vi "AnnularArraySIR.vi"(0 "Trans Geometry":T5={"ROC (cm)"=1.2, "a (cm)"=0.3, "focus location"=1.2} {"focus location" format="%.2f"; "a (cm)" format="%.2f"; "ROC (cm)" format="%.2f"}, 1 "Pressure Calc":u16(ring)=1 items=["Pos Peak", "Neg peak", "Pk-Pk", "Steady State", "CW Drive", "Pii"], 3 "center of calc":dbl, 4 "Save Options":T3={"Save h Files?"=FALSE, "Save image data?"=FALSE, "Path"=path "F:/Test"}, 5 "Center Hole":dbl format="%.2f", 6 "Recip Processing":u16[][](array[ring])=[[1, 1, 1, 1, 1], [1, 1, 1, 1, 1], [1, 1, 1, 1, 1], [1, 1, 1, 1, 1], [1, 1, 1, 1, 1]] items=["0", "1", "2"], 7 "Wave Source":T1={"Load Wave File"=FALSE, "file path"=path "F:/PVDFXducer/FiveRing/5Ring5/83micH/R1quartz.txt", "Up sample fac"=1}, 8 "Variables":T6={"Number of rings"=5, "sound spd (cm/s)"=150000, "z span (cm)"=0.1, "z steps"=11, "y span (cm)"=0.05, "y steps"=30, "time step (s)"=1e-10, "z"=0.0, "y"=0.0, "ref delay"=0.0, "freq (MHz)"=4.5, "cycles"=5.0} {"freq (MHz)" format="%.2f"; "z span (cm)" format="%.2f"; "y" format="%.2f"; "ref delay" format="%.2f"; "y span (cm)" format="%.4f"; "z" format="%.2f"; "time step (s)" format="%.2e"}, 10 "Calc":u16(ring) items=["One way", "RT Single Rings", "R/T Full Aperture", "Time Domain PSF"], 11 "DR Inputs":T2 {"Tansducer" items=["F2 40 MHz", "F3 20 MHz"]}, 12 "Active Annuli":bool[](array[boolean]), 13 "kerf space (cm)":dbl=0.01 format="%.5f") -> (14 "Output Data":T4 {"pressures" format="%.2f"; "y-axis" format="%.2f"; "z-axis" format="%.2f"}, 19 "time data out":dbl[][](array[numeric]))   [LabVIEW 2022 SP3]
uses:
  <vilib>/Math Plots/3D Math Plots/3D Surface/3D Surface XCtrl/3D Surface.xctl
  <vilib>/Analysis/2dsp.llb/Decimate (single shot, DBL).vi
  <vilib>/Math Plots/3D Math Plots/3D Surface/3D Surface Datatype/Public/Plot Helper (Vector).vi
  <vilib>/Utility/file.llb/Write Delimited Spreadsheet (DBL).vi
  <vilib>/Utility/file.llb/Write To Spreadsheet File (DBL).vi
  <vilib>/Analysis/NI_AALBase.lvlib
  <vilib>/Analysis/NI_AALPro.lvlib
  <vilib>/Math Plots/3D Math Plots/3D Surface/3D Surface Datatype/3D Surface Datatype.lvclass
panel:
  out "3D Surface":refnum<class "3D Plot Datatype.lvclass">[](xcontrol)
  out "data out":sgl[][][](array[numeric])
  out "Waveform Graph":dbl[](graph)
  out "max value":dbl
  in  "norm ?":bool
  in  "Gain":dbl[](array[numeric]) format="%.2f"
  in  "Kerf?":bool=TRUE
  out "3 dB beamwidth axial":dbl format="%.4f"
  in  "SAVE DATA?":bool
  out "oneil axial P":cluster{dbl[], "Y[i]=X[i]/Max|X|":dbl[]}(graph)
  in  "full h(r,t)?":bool
  in  "Number of rings":i32=-1
  in  "Make Report":bool
  out "axial peak (cm)":dbl format="%.2f"
  out "3 dB beamwidth (cm)":dbl format="%.4f"
  out "lateral pressure":cluster{"output":dbl[], "output":dbl[]}(graph)
  out "Rings":picture
  out "axial pressure":cluster{dbl[], "output":dbl[]}(graph)
  # "Quantel Probe\n0 1.895 1.995 2.75 2.85 3.42  3.52  3.99 4.09  4.5 \ngeometricFocusMm=23.2"
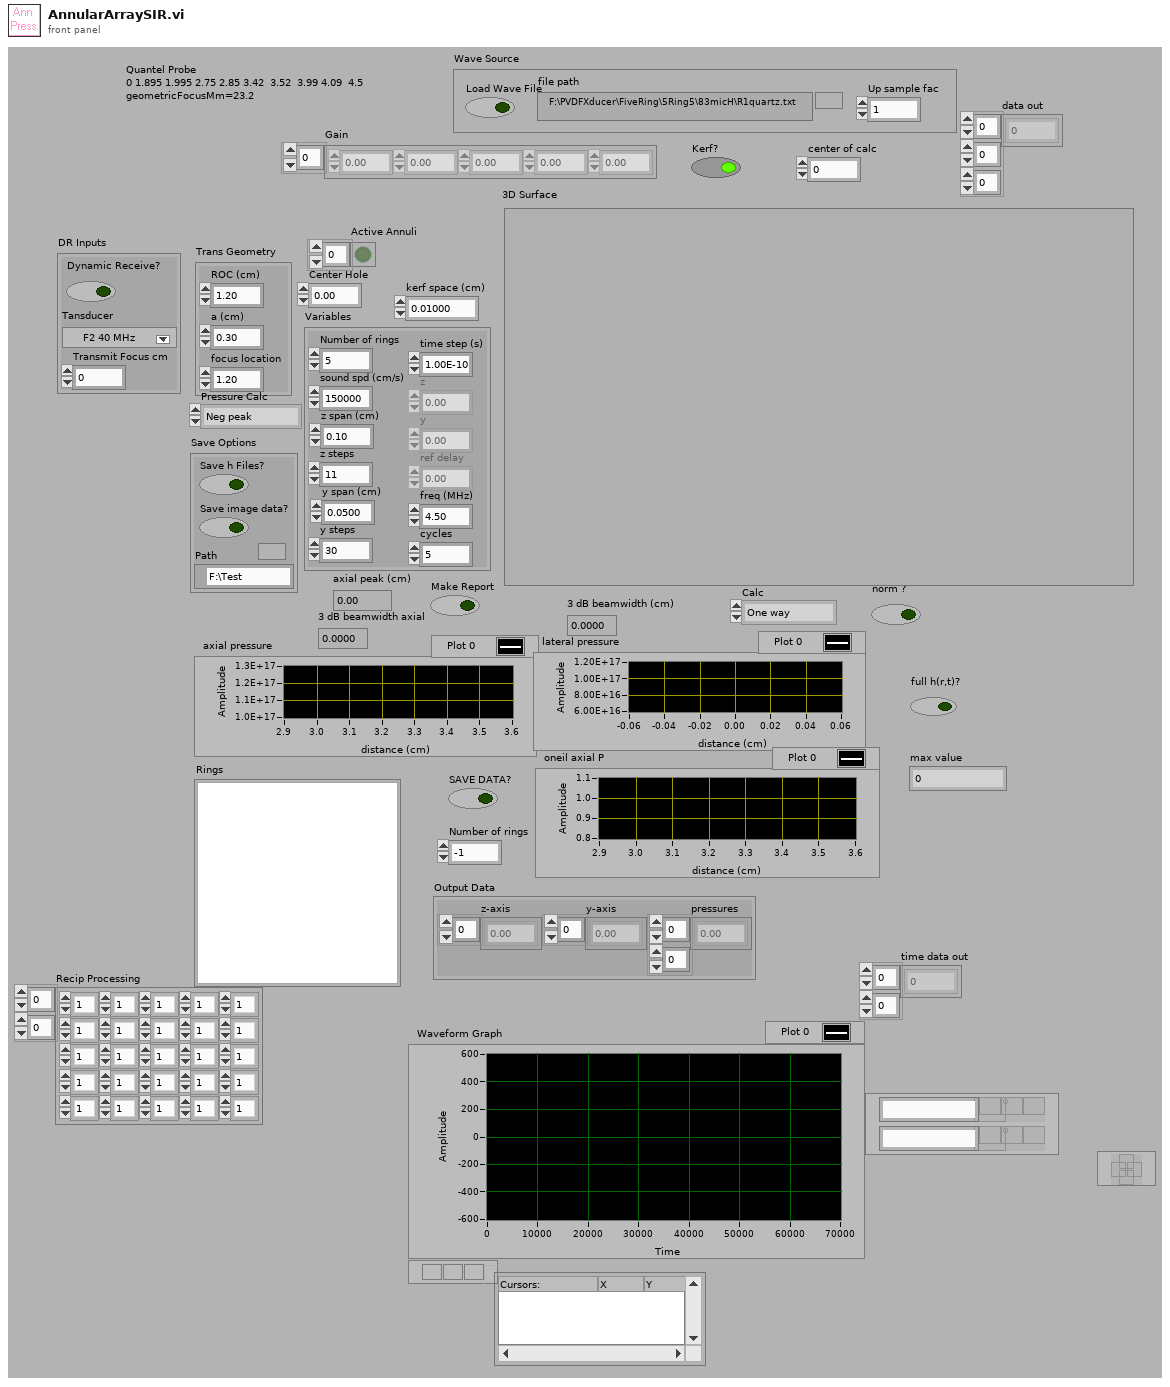
[diagram p1: front panel]
types:
  T1 = cluster{"Load Wave File":bool, "file path":path, "Up sample fac":i32}
  T2 = cluster{"Dynamic Receive?":bool, "Tansducer":u16, "Transmit Focus cm":dbl}
  T3 = cluster{"Save h Files?":bool, "Save image data?":bool, "Path":path}
  T4 = cluster{"z-axis":dbl[], "y-axis":dbl[], "pressures":dbl[][]}
  T5 = cluster{"ROC (cm)":dbl, "a (cm)":dbl, "focus location":dbl}
  T6 = cluster{"Number of rings":i32, "sound spd (cm/s)":i32, "z span (cm)":dbl, "z steps":i32, "y span (cm)":dbl, "y steps":i32, "time step (s)":sgl, "z":dbl, "y":dbl, "ref delay":dbl, "freq (MHz)":dbl, "cycles":sgl}
  T7 = cluster{"Annular rings":cluster{"Radius":dbl, "a":dbl}[], "Waveform":dbl[], "focus delay abs (s)":dbl}[]
  T8 = cluster{"Number of rings":i32, "sound spd (cm/s)":i32, "z span (cm)":dbl, "z steps":i32, "y spacing (cm)":dbl, "y steps":i32, "time step (s)":sgl, "z":dbl, "y":dbl, "ref delay":dbl, "freq (MHz)":dbl, "cycles":sgl}
  T9 = cluster{dbl[], "output":dbl[], "Yij=Xij/Max|X|":dbl[][]}
  T10 = cluster{"axial pressure (z)":cluster{dbl[], "output":dbl[]}, "3 dB beamwidth (cm)":dbl, "lateral pressure (y)":cluster{"output":dbl[], "output":dbl[]}, "3 dB beamwidth (cm)":dbl}
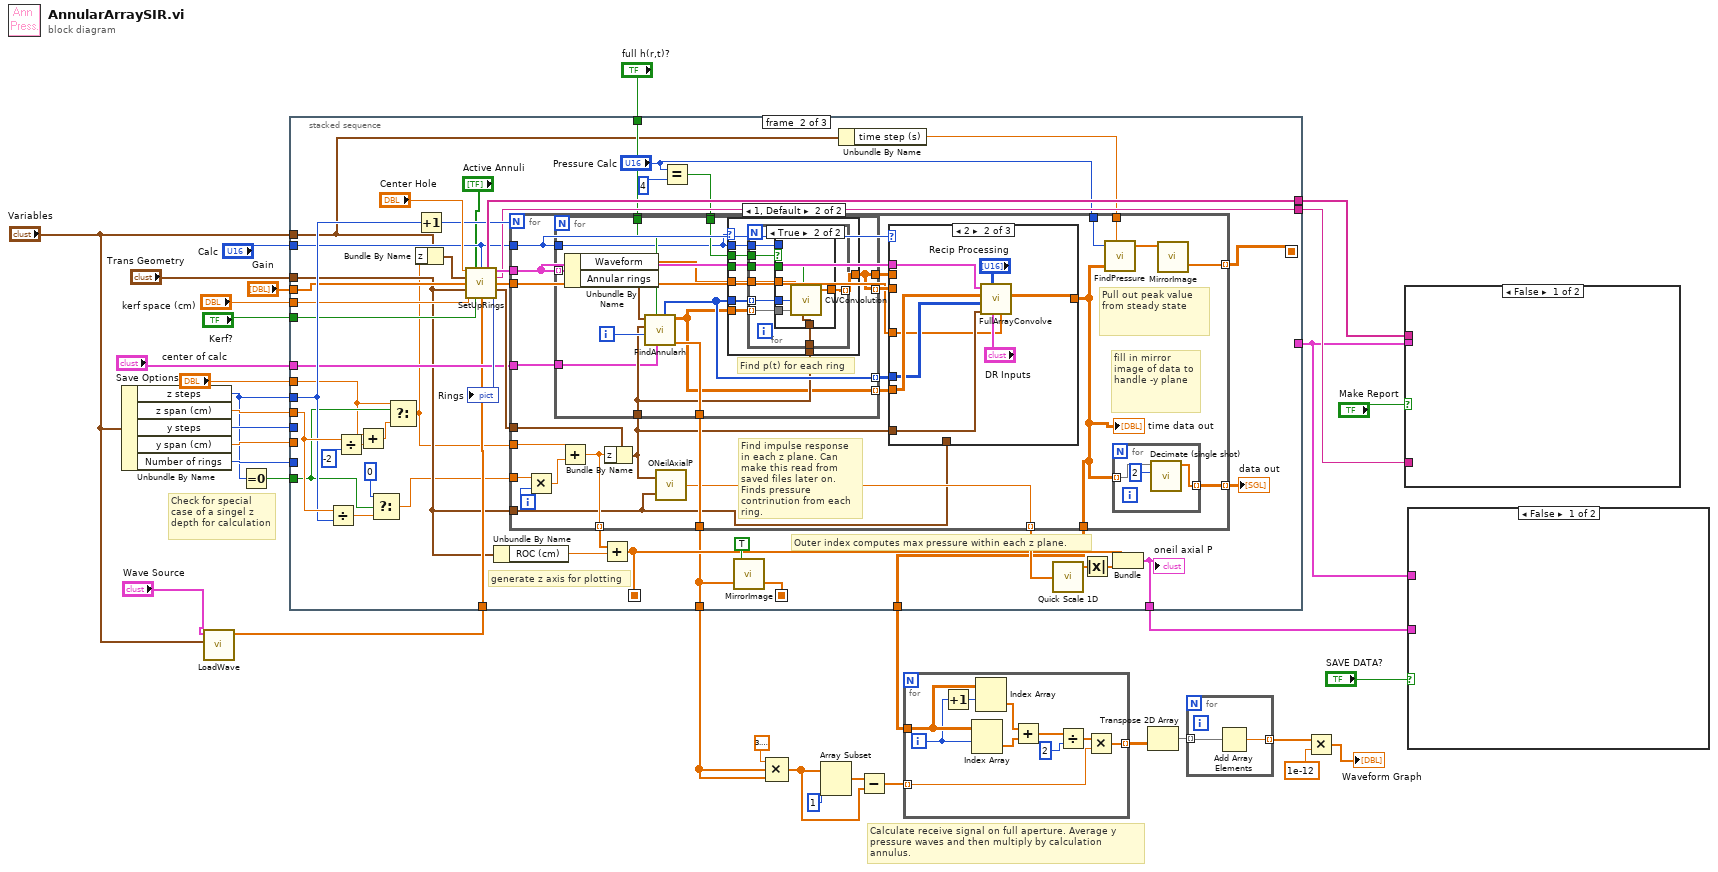
[diagram p0: block diagram]
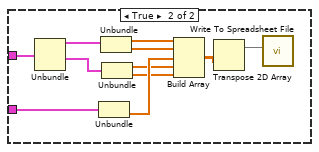
[diagram p2: hidden frame]
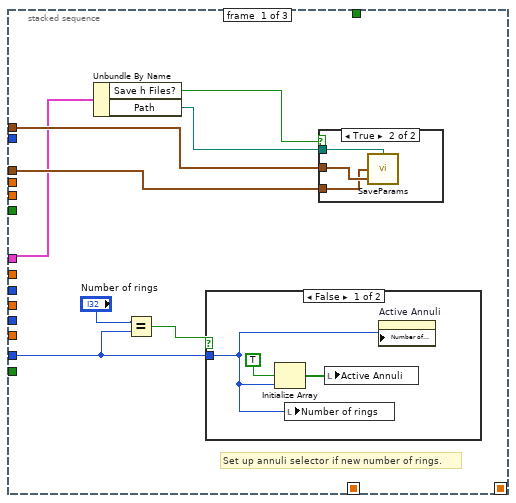
[diagram p3: hidden frame]
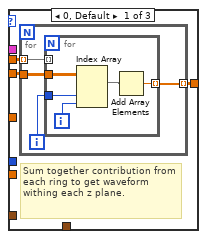
[diagram p6: hidden frame]
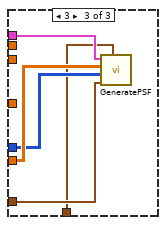
[diagram p7: hidden frame]
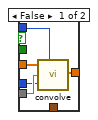
[diagram p9: hidden frame]
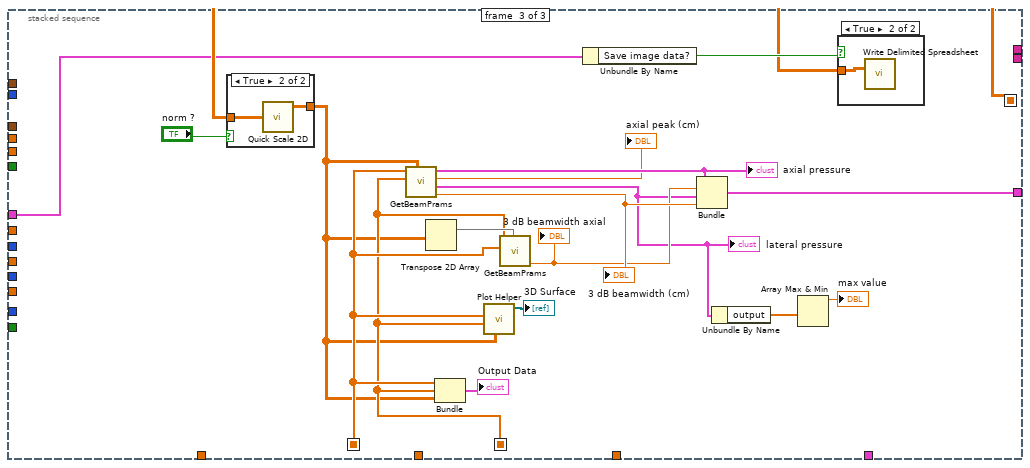
[diagram p10: hidden frame]
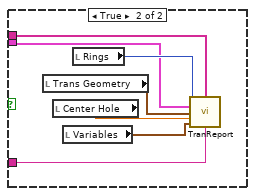
[diagram p13: hidden frame]
diagram:
  # "Calculate receive signal on full aperture. Average y pressure waves and then multiply by calculation annulus."
  # "Check for special case of a singel z depth for calculation"
  n1 = Unbundle By Name("Variables") -> ("z steps"=w17:i32, "z span (cm)"=w35:dbl, "y steps"=w30:i32, "y span (cm)"=w29:dbl, "Number of rings"=w32:i32)
  n2 = call "LoadWave.vi"("Variables"="Variables", "Wave Source"="Wave Source") -> ("Waveform Graph"=w1:dbl[])  [unwired: 1 in, 8 out]
  n3 = Equal To 0?(x=w17) -> (x = 0?=w16:bool)
  n4 = stacked-sequence {
    seq-local: [_ w77 _] -> [_ _ w200]
    seq-local: [_ w84 _] -> [_ _ w192]
    seq-local: [_ w74 _] -> [_ _ w193]
    tunnel: w35 -> [_ w92 _]
    tunnel: "Save Options" -> [w36 w87 w195]
    tunnel: "Trans Geometry" -> [w42 w67 _]
    tunnel: "Variables" -> [w43 w57 _]
    tunnel: w17 -> [_ w88 _]
    tunnel: w32 -> [w38 _ _]
    tunnel: w30 -> [_ _ _]
    tunnel: w29 -> [_ _ _]
    tunnel: [_ _ w207] -> w25
    tunnel: [_ w83 _] -> w28
    tunnel: [_ w81 _] -> w26
    tunnel: "full h(r,t)?" -> [_ w78 _]
    tunnel: [_ w72 _] -> w24
    tunnel: "kerf space (cm)" -> [_ w71 _]
    tunnel: "Kerf?" -> [_ w70 _]
    tunnel: w1 -> [_ w69 _]
    tunnel: "Gain" -> [_ w68 _]
    tunnel: "Calc" -> [_ w66 _]
    tunnel: "center of calc" -> [_ w50 _]
    tunnel: w16 -> [_ w59 _]
    tunnel: [_ w54 _] -> w8
    tunnel: [_ w52 _] -> w2
    frame #0 {
      # "Set up annuli selector if new number of rings."
      n5 = Unbundle By Name(w36) -> ("Save h Files?"=w40:bool, "Path"=w41:path)
      n6 = Equal?(x="Number of rings", y=w38) -> (x = y?=w37:bool)
      n7 = case shown="False" w37 {
        tunnel: w38 -> [w45 _]
        frame False {
          n8 = Initialize Array(TRUE, w45) -> (w44:bool[])
          n9 = local write "Number of rings"(w45) -> ()
          n10 = local write "Active Annuli"(w44) -> ()
          n11 = property on="Active Annuli" class="Arr (strict)"("Number of Columns"=w45) -> ()  [unwired: 2 in, 2 out]
        }
        frame True {
        }
      }
      n12 = case shown="True" w40 {
        tunnel: w41 -> [_ w49]
        tunnel: w43 -> [_ w48]
        tunnel: w42 -> [_ w47]
        frame False {
        }
        frame True {
          n13 = call "SaveParams.vi"("Variables"=w48, "Trans Geometry"=w47, "Path"=w49) -> ()
        }
      }
    }
    frame #1 {
      # "generate z axis for plotting"
      # "Outer index computes max pressure within each z plane."
      n14 = Divide(x=w92, y=w88) -> (x/y=w63:dbl)
      n15 = Divide(x=w92, y=-2) -> (x/y=w60:dbl)
      n16 = Add(x=w50, y=w60) -> (x+y=w64:dbl)
      n17 = Select(t=0, s=w59, f=w63) -> (s? t:f=w61:dbl)
      n18 = Select(t=w50, s=w59, f=w64) -> (s? t:f=w65:dbl)
      n19 = Increment(x=w88) -> (x+1=w82:i32)
      n20 = Bundle By Name(cluster=w57, "z"=w65) -> (w94:T6)
      n21 = call "SetUpRings.vi"("Center Hole"="Center Hole", "Array"="Active Annuli", "Calc"=w66, "Variables"=w94, "Gain"=w68, "Trans Geometry"=w67, "kerf space (cm)"=w71, "Kerf?"=w70, "Drive waveform"=w69) -> ("annuli list"=w83:string[], 4:"Rings"=w95:T7, "projected ring locations"=w81:string, "rings (m)"=w58:dbl[], "Variables out"=w91:T8, 15:"Rings"=→"Rings":picture)  [unwired: 1 in]
      n22 = Unbundle By Name(w67) -> ("ROC (cm)"=w85:dbl)
      n23 = Equal?(x="Pressure Calc", y=4) -> (x = y?=w79:bool)
      n24 = Unbundle By Name(w57) -> ("time step (s)"=w56:sgl)
      n25 = for {
        N: w82 -> [_]
        tunnel: w95 -> [w104]
        tunnel: w65 -> [w117]
        tunnel: w61 -> [w120]
        tunnel: [w113] -> w77 mode=indexing
        tunnel: w91 -> [w118]
        tunnel: [w116] -> w54
        tunnel: "Pressure Calc" -> [w115]
        tunnel: [w112] -> w86 mode=indexing
        tunnel: w87 -> [w111]
        tunnel: w79 -> [w110]
        tunnel: w78 -> [w109]
        tunnel: w67 -> [w97]
        tunnel: [w108] -> w76 mode=indexing
        tunnel: w66 -> [w102]
        tunnel: w58 -> [w101]
        tunnel: w56 -> [w100]
        tunnel: [w99] -> w53 mode=indexing
        tunnel: [w98] -> w52
        i -> [w121]
        # "fill in mirror image of data to handle -y plane"
        # "Pull out peak value from steady state"
        # "Find impulse response in each z plane. Can make this read from saved files later on. Finds pressure contrinution from each ring."
        n26 = Multiply(x=w120, y=w121) -> (x*y=w122:dbl)
        n27 = Add(x=w117, y=w122) -> (x+y=w112:dbl)
        n28 = Bundle By Name(cluster=w118, "z"=w112) -> (w103:T8)
        n29 = for {
          tunnel: w103 -> [w156]
          tunnel: w104 -> [w161] mode=indexing
          tunnel: [w158] -> w107 mode=indexing
          tunnel: [w158] -> w119
          tunnel: [w163] -> w116
          tunnel: w111 -> [w154]
          tunnel: w110 -> [w162]
          tunnel: w109 -> [w160]
          tunnel: w102 -> [w152]
          tunnel: [w159] -> w106 mode=indexing
          tunnel: [w153] -> w105 mode=indexing
          i -> [w157]
          # "Find p(t) for each ring"
          n30 = Unbundle By Name(w161) -> ("Waveform"=w151:dbl[], "Annular rings"=w155:cluster{"Radius":dbl, "a":dbl}[])
          n31 = call "FindAnnularh.vi"("Save Options"=w154, "Full h(r,t)"=w160, "Ring Number"=w157, "Variables in"=w156, "Annular rings"=w155) -> ("Y axis"=w163:dbl[], "h(r,t)"=w153:dbl[][], "delay pts"=w159:i32[])  [unwired: 4 in]
          n32 = case shown="1, Default" w152 {
            tunnel: [_ w171] -> w158
            tunnel: w151 -> [_ w170]
            tunnel: w162 -> [_ w169]
            tunnel: w156 -> [_ w168]
            tunnel: w160 -> [_ w167]
            tunnel: w152 -> [_ w166]
            tunnel: w159 -> [_ w165]
            tunnel: w153 -> [_ w164]
            frame 2, 3 {
            }
            frame 1, Default {
              n33 = for {
                tunnel: w164 -> [w179] mode=indexing
                tunnel: w170 -> [w176]
                tunnel: [w178] -> w171 mode=indexing
                tunnel: w169 -> [w177]
                tunnel: w168 -> [w175]
                tunnel: w165 -> [w173] mode=indexing
                tunnel: w167 -> [w174]
                tunnel: w166 -> [w172]
                n34 = case shown="True" w177 {
                  tunnel: w179 -> [w184 w187]
                  tunnel: w176 -> [w183 w189]
                  tunnel: [w182 w190] -> w178
                  tunnel: w175 -> [_ w188]
                  tunnel: w173 -> [w181 w186]
                  tunnel: w174 -> [_ w185]
                  tunnel: w172 -> [w180 _]
                  frame False {
                    n35 = call "convolve.vi"("X"=w183, "Calc"=w180, "Y"=w184, "delay pts"=w181) -> ("X*Y"=w182:dbl[])  [unwired: 2 out]
                  }
                  frame True {
                    n36 = call "CWConvolution.vi"("delay waveform"=w189, "Boolean"=w185, "delay pts"=w186, "h(r,t)"=w187, "Variables"=w188) -> ("X*Y"=w190:dbl[])  [unwired: 2 out]
                  }
                }
              }
            }
          }
        }
        n37 = call "ONeilAxialP.vi"("Trans Geometry"=w97, "Variables"=w103) -> ("Output Variable"=w108:dbl)
        n38 = case shown="2" w102 {
          tunnel: w119 -> [w128 _ _]
          tunnel: [w127 w139 _] -> w98
          tunnel: w107 -> [w126 _ _]
          tunnel: w106 -> [_ w144 w149]
          tunnel: w105 -> [_ w145 w150]
          tunnel: w104 -> [_ w143 w148]
          tunnel: w103 -> [_ w142 w147]
          tunnel: w101 -> [_ w140 _]
          tunnel: w97 -> [_ _ w146]
          frame 0, Default {
            # "Sum together contribution from each ring to get waveform withing each z plane."
            n39 = for {
              tunnel: w126 -> [w132]
              tunnel: [w129] -> w127 mode=indexing
              tunnel: w128 -> [w130] mode=indexing
              i -> [w131]
              n40 = for {
                tunnel: w132 -> [w137]
                tunnel: w131 -> [w135]
                tunnel: [w134] -> w129 mode=indexing
                tunnel: w130 -> [_] mode=indexing
                i -> [w136]
                n41 = Index Array(array=w137, index (dim 1)=w135, index (dim 2)=w136) -> (element=w133:dbl[])  [unwired: 1 in]
                n42 = Add Array Elements(numeric array=w133) -> (sum=w134:dbl)
              }
            }
          }
          frame 2 {
            n43 = call "FullArrayConvolve.vi"("rings"=w140, "DR Inputs"="DR Inputs", "Recip Processing"="Recip Processing", "Variables"=w142, "delay pts"=w144, "h(r,t)"=w145, "Rings"=w143) -> ("data out"=w139:dbl[][])  [unwired: 4 out]
          }
          frame 3 {
            n44 = call "GeneratePSF.vi"("Trans Geometry"=w146, "Variables"=w147, "delay pts"=w149, "h(r,t)"=w150, "Rings"=w148) -> ()  [unwired: 7 in]
          }
        }
        "time data out" <- w98
        n45 = call "FindPressure.vi"("Pressure Calc"=w115, "time step (s)"=w100, "Input"=w98) -> ("Pressures"=w114:dbl[])  [unwired: 4 out]
        n46 = for {
          tunnel: w98 -> [w125] mode=indexing
          tunnel: [w124] -> w99 mode=indexing
          n47 = call-poly <vilib>:"Decimate (single shot).vi"("decimating factor"=2, "X"=w125) -> ("Decimated Array"=w124:dbl[])  [unwired: 8 in, 1 out]
        }
        n48 = call "MirrorImage.vi"("input"=w114) -> ("output"=w113:dbl[])  [unwired: 1 in, 1 out]
      }
      "data out" <- w53
      n49 = Add(x=w86, y=w85) -> (x+y=w74:dbl[])
      n50 = call "MirrorImage.vi"("input"=w54, "neg?"=TRUE) -> ("output"=w84:dbl[])  [unwired: 1 out]
      n51 = call <vilib>:"Quick Scale 1D.vi"("X"=w76) -> ("Y[i]=X[i]/Max|X|"=w75:dbl[])  [unwired: 2 out]
      n52 = Absolute Value(x=w75) -> (abs(x)=w73:dbl[])
      n53 = Bundle(w74, w73) -> (w72:cluster{dbl[], dbl[]})  [unwired: 1 out]
      "oneil axial P" <- w72
    }
    frame #2 {
      n54 = case shown="True" "norm ?" {
        tunnel: w200 -> [w209 w211]
        tunnel: [w209 w210] -> w191
        frame False {
        }
        frame True {
          n55 = call <vilib>:"Quick Scale 2D.vi"("X"=w211) -> ("Yij=Xij/Max|X|"=w210:dbl[][])  [unwired: 2 out]
        }
      }
      n56 = call "GetBeamPrams.vi"("data"=w191, "ycoords"=w192, "x coords"=w193) -> ("3 dB beamwidth (cm)"=w204:dbl, "lateral pressure (y)"=w198:cluster{"output":dbl[], "output":dbl[]}, "axial peak (cm)"=→"axial peak (cm)":dbl, "axial pressure (z)"=w205:cluster{dbl[], "output":dbl[]})  [unwired: 1 in, 1 out]
      "3 dB beamwidth (cm)" <- w204
      "lateral pressure" <- w198
      "axial pressure" <- w205
      n57 = Transpose 2D Array(2D array=w191) -> (transposed array=w203:dbl[][])
      n58 = Bundle(w193, "output"=w192, "Yij=Xij/Max|X|"=w191) -> (→"Output Data":T9)  [unwired: 1 out]
      n59 = call-poly <vilib>:"Plot Helper.vi"("z matrix"=w191, "y vector"=w192, "x vector"=w193) -> ("3D Plot lvclass Array out"=→"3D Surface":refnum<class "3D Plot Datatype.lvclass">[])  [unwired: 3 in, 5 out]
      n60 = call "GetBeamPrams.vi"("data"=w203, "ycoords"=w193, "x coords"=w192) -> ("3 dB beamwidth (cm)"=w201:dbl)  [unwired: 1 in, 4 out]
      "3 dB beamwidth axial" <- w201
      n61 = Unbundle By Name(w195) -> ("Save image data?"=w206:bool)
      n62 = Bundle("axial pressure (z)"=w205, "3 dB beamwidth (cm)"=w201, "lateral pressure (y)"=w198, "3 dB beamwidth (cm)"=w204) -> (w207:T10)  [unwired: 1 out]
      n63 = Unbundle By Name(w198) -> ("output"=w197:dbl[])
      n64 = Array Max & Min(array=w197) -> (max value=→"max value":dbl)  [unwired: 3 out]
      n65 = case shown="True" w206 {
        tunnel: w200 -> [_ w212]
        frame False {
        }
        frame True {
          n66 = call-poly <vilib>:"Write Delimited Spreadsheet.vi"("2D data"=w212) -> ()  [unwired: 13 in, 2 out]
        }
      }
    }
  }
  n67 = Compound Arithmetic op=MULTIPLY(3.141592653589793, w8, w8) -> (w9:dbl[])
  n68 = Array Subset(array=w9, index=1) -> (w10:dbl[])  [unwired: 1 in]
  n69 = Subtract(x=w10, y=w9) -> (x-y=w7:dbl[])
  n70 = for {
    tunnel: w2 -> [w222]
    tunnel: [w213] -> w6 mode=indexing
    tunnel: w7 -> [w214] mode=indexing
    i -> [w220]
    n71 = Increment(x=w220) -> (x+1=w221:i32)
    n72 = Index Array(array=w222, index (row)=w220) -> (element=w218:dbl[])  [unwired: 1 in]
    n73 = Index Array(array=w222, index (row)=w221) -> (element=w219:dbl[])  [unwired: 1 in]
    n74 = Add(x=w219, y=w218) -> (x+y=w217:dbl[])
    n75 = Divide(x=w217, y=2) -> (x/y=w215:dbl[])
    n76 = Multiply(x=w215, y=w214) -> (x*y=w213:dbl[])
  }
  n77 = Transpose 2D Array(2D array=w6) -> (transposed array=w13:dbl[][])
  n78 = for {
    tunnel: w13 -> [w224] mode=indexing
    tunnel: [w223] -> w5 mode=indexing
    n79 = Add Array Elements(numeric array=w224) -> (sum=w223:dbl)
  }
  n80 = Multiply(x=w5, y=1e-12) -> (x*y=→"Waveform Graph":dbl[])
  n81 = case shown="False" "Make Report" {
    tunnel: w25 -> [_ w227]
    tunnel: w28 -> [_ w226]
    tunnel: w26 -> [_ w225]
    frame False {
    }
    frame True {
      n82 = local read "Trans Geometry"() -> (w230:T5)
      n83 = local read "Center Hole"() -> (w231:dbl)
      n84 = local read "Variables"() -> (w229:T6)
      n85 = local read "Rings"() -> (w228:picture)
      n86 = call "TranReport.vi"("Rings"=w228, "annuli list"=w226, "Output Cluster"=w227, "Trans Geometry"=w230, "Center Hole"=w231, "Variables"=w229, "ring locations"=w225) -> ()  [unwired: 2 in, 7 out]
    }
  }
  n87 = case shown="False" "SAVE DATA?" {
    tunnel: w25 -> [_ w242]
    tunnel: w24 -> [_ w239]
    frame False {
    }
    frame True {
      n88 = Unbundle(w242) -> ("axial pressure (z)"=w241:cluster{dbl[], "output":dbl[]}, "lateral pressure (y)"=w240:cluster{"output":dbl[], "output":dbl[]})  [unwired: 2 out]
      n89 = Unbundle(w239) -> (w236:dbl[])  [unwired: 1 out]
      n90 = Unbundle(w241) -> (w238:dbl[], "output"=w237:dbl[])
      n91 = Unbundle(w240) -> ("output"=w235:dbl[], "output"=w234:dbl[])
      n92 = Build Array(w238, w237, w236, w235, w234) -> (w233:dbl[][])
      n93 = Transpose 2D Array(2D array=w233) -> (transposed array=w232:dbl[][])
      n94 = call-poly <vilib>:"Write To Spreadsheet File.vi"("2D data"=w232) -> ()  [unwired: 5 in, 3 out]
    }
  }
